vi "PH_Sequencer.PC CheckTOs.vi"(0 "i ref in":refnum<vi>, 5 "error in (no error)":errorcluster) -> (14 "i ref out":refnum<vi>, 19 "error out":errorcluster)   [LabVIEW 2014, in "PH_Sequencer.lvlib"]
doc: "This VI checks whether a timeout occured. It writes this information to own attributes and indicates it on the GUI."
uses:
  PH_Sequencer.lvlib
  PH_Basics/PH_PowerUnit_BaseClass/PH_PowerUnit_BaseClass.SM States.ctl
  PH_Basics/PH_Common/PH_Common.lvlib
  PH_Basics/PH_PowerUnit_BaseClass/PH_PowerUnit_BaseClass.lvlib
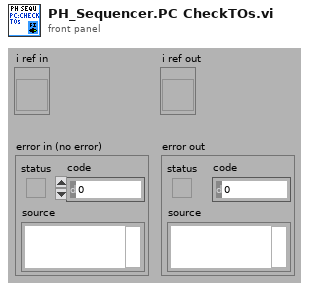
[diagram p1: front panel]
types:
  T1 = typedef "PH_Sequencer.lvlib/PH_Sequencer.i attribute.ctl" = cluster{"GUI Refs":cluster{"Main Off":refnum<vi>, "Fire":refnum<vi>, "Status":refnum<vi>, "Ready":refnum<vi>, "Waiting Time":refnum<vi>, "Timeout":refnum<vi>, "PPMA Ready":refnum<vi>, "Sequencer SM State":refnum<vi>, "PPPA Ready":refnum<vi>, "Calorimeter":refnum<vi>, "Beamline Ready":refnum<vi>, "Clear Beamline":refnum<vi>, "Linkage PPMA Rods":refnum<vi>, "Linkage Current PA":refnum<vi>, "Linkage Current MA":refnum<vi>, "Timing Ready":refnum<vi>, "State Timing":refnum<vi>, "Force Timing":refnum<vi>, "PSDB Shot Comment":refnum<vi>, "State PA Backreflection":refnum<vi>, "Beamline Z6 Ready":refnum<vi>, "Clear Z6 Beamline":refnum<vi>, "Sequence length":refnum<vi>, "Timing Mode":refnum<vi>, "Slow Trigger Settings":refnum<vi>, "Experiment Description":refnum<vi>, "State PSDB":refnum<vi>, "PSDB Ready":refnum<vi>, "Set PSDB Settings":refnum<vi>, "Get PSDB Info":refnum<vi>, "Take Snapshot":refnum<vi>, "Shottype":refnum<vi>, "Experiment":refnum<vi>, "Phase Frontends":refnum<vi>, "PP 45mm PILC in use":refnum<vi>}, "Status Info":cluster{"Machine Status":T2, "WaitingTime":i32, "Timeout":bool}, "Readyness":cluster{"Ready to shot":bool, "PPMA Ready":bool, "PPPA Ready":bool, "BL Ready":bool, "Timing Ready":bool, "BL Z6 Ready":bool, "PSDBReady":bool}, "Instancenames":cluster{"PPMA Rods":string, "PP Current Meas":string, "PH Beamline Chief":string, "PA Backrefl Meas":string, "Z6 Beamline Chief":string}, "Data to read":bool, "Calorimeter":cluster{"Instancename":string, "On":bool, "linked":bool}, "Linkage":cluster{"PPMA Rods":bool, "PP Current Meas":bool, "PHELIX Beamline Chief":bool, "PA Backrefl Meas":bool, "Z6 Beamline Chief":bool}, "Timing":cluster{"Instance":string, "linked":bool, "Status":T2, "Timing Mode":T3, "Slow Trigger Settings":T4, "Info available":cluster{"ext SlowTrigger":bool, "T2":bool, "Mode":bool, "Delay Slow Trigger":bool, "Phase FEs":bool}, "FE Phase":T5}, "Service ID R2S":i32, "PSDB":cluster{"Controller Instance":string, "Controller Status":T2, "Controller linked":bool, "Settings acknowledged":bool, "Current Experiment ID":i16, "Current Shot Type":i16, "Current Comment":string, "Remember Settings":bool, "Write 2 early":bool}, "PSDB Data":cluster{"Main Off?":bool, "Sequence Length":dbl, "Sequence startet":timestamp}, "6P 4Q Positions":cluster{"Instancename":string, "linked":bool, "Position":T6}[], "PUs":T7[]}
  T2 = typedef "PH_StatusHandler.lvlib/PH_StatusHandler.Status.ctl" = i16
  T3 = typedef "PH_Timing.lvlib/PH_Timing.Timing Mode.ctl" = cluster{"T2":i16, "Modeselector":enum32{"10 Hz", "0.5 Hz", "Shot"}}
  T4 = typedef "PH_Timing.lvlib/PH_Timing.Slow Trigger Settings.ctl" = cluster{"Delay":dbl, "externally triggered?":bool}
  T5 = typedef "PH_Timing.lvlib/PH_Timing.Phase FEs.ctl" = cluster{"Phase":dbl}
  T6 = typedef "PH_4_Pos_Selector.lvlib/PH_4_Pos_Selector.Position Selector.ctl" = u16
  T7 = typedef "PH_Sequencer.lvlib/PH_Sequencer.Head.ctl" = cluster{"PowerUnit":T8, "GUI Ref":refnum<vi>, "Information":T9, "linked?":bool, "GUI Ref Current Voltage":refnum<vi>}
  T8 = typedef "PH_PP_Common.lvlib/PH_PP_Common.PUs.ctl" = enum16{"no Info", "PA-19mm-1", "PA-19mm-2", "PA-45mm-PILC", "PA-45mm-MAIN", "MA-PU-1", "MA-PU-2", "MA-PU-3", "MA-PU-4", "MA-PU-5", "MA-PU-6", "MA-FR", "MA-PILC", "PA-45mm-DP"}
  T9 = typedef "PH_Sequencer.lvlib/PH_Sequencer.PU Information.ctl" = cluster{"State":T2, "Waiting Time [s]":dbl, "PU State SM":T10, "PU Timeout SM":T10}
  T10 = typedef "PH_PowerUnit_BaseClass.lvlib/PH_PowerUnit_BaseClass.SM States.ctl" = enum16{".", "Stand by", "Switch PU on", "Configure", "Set Default Voltage", "Set STANDBY", "Set READY", "Wait for Shot Cmd", "Open Dump Rods", "Open Ross Relais", "Close Ross Relais", "Switch PSU on", "Switch PSU off", "Charge", "Switch GD Channel on", "Close Dump Rods", "Rods-TO", "RR-TO", "PSU-TO", "Trigger-TO"}
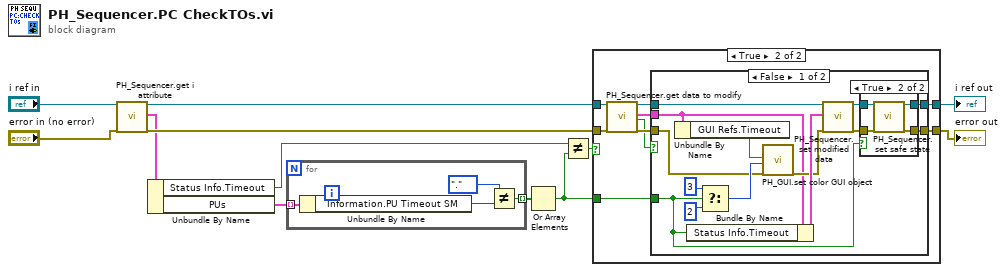
[diagram p0: block diagram]
diagram:
  n1 = call "PH_Sequencer.get i attribute.vi"("i ref in"="i ref in", "error in (no error)"="error in (no error)") -> ("i ref out"=w11:refnum<vi>, "i attribute"=w8:T1, "error out"=w9:errorcluster)  [unwired: 15 in]
  n2 = Unbundle By Name(w8) -> ("Status Info.Timeout"=w4:bool, "PUs"=w2:T7[])
  n3 = for {
    tunnel: w2 -> [w15] mode=indexing
    tunnel: [w16] -> w1 mode=indexing
    n4 = Unbundle By Name(w15) -> ("Information.PU Timeout SM"=w14:T10)
    n5 = Not Equal?(x=PH_PowerUnit_BaseClass.SM_States.".", y=w14) -> (x != y?=w16:bool)
  }
  n6 = Or Array Elements(Boolean array=w1) -> (logical OR=w3:bool)
  n7 = Not Equal?(x=w4, y=w3) -> (x != y?=w5:bool)
  n8 = case shown="True" w5 {
    tunnel: [w18 w27] -> w12
    tunnel: w11 -> [w18 w26]
    tunnel: [w17 w25] -> w10
    tunnel: w9 -> [w17 w24]
    tunnel: w3 -> [_ w23]
    frame False {
    }
    frame True {
      n9 = call "PH_Sequencer.get data to modify.vi"("i ref in"=w26, "error in (no error)"=w24) -> ("i ref out"=w21:refnum<vi>, "i attribute"=w20:T1, "timed out"=w19:bool, "error out"=w22:errorcluster)  [unwired: 14 in]
      n10 = case shown="False" w19 {
        tunnel: [w41 w49] -> w27
        tunnel: [w40 w48] -> w25
        tunnel: w23 -> [w35 _]
        tunnel: w22 -> [w31 w48]
        tunnel: w21 -> [w30 w49]
        tunnel: w20 -> [w29 _]
        frame False {
          n11 = Unbundle By Name(w29) -> ("GUI Refs.Timeout"=w28:refnum<vi>)
          n12 = Bundle By Name(cluster=w29, "Status Info.Timeout"=w35) -> (w39:T1)
          n13 = Select(t=3, s=w35, f=2) -> (s? t:f=w34:i32)
          n14 = call "PH_GUI.set color GUI object.vi"("GUI object Ref"=w28, "State"=w34, "error in (no error)"=w31) -> ("error out"=w33:errorcluster)  [unwired: 16 in]
          n15 = call "PH_Sequencer.set modified data.vi"("i ref in"=w30, "i attribute"=w39, "error in (no error)"=w33) -> ("i ref out"=w38:refnum<vi>, "error out"=w37:errorcluster)  [unwired: 15 in]
          n16 = case shown="True" w35 {
            tunnel: w38 -> [w43 w44]
            tunnel: [w43 w47] -> w41
            tunnel: w37 -> [w42 w46]
            tunnel: [w42 w45] -> w40
            frame False {
            }
            frame True {
              n17 = call "PH_Sequencer.set safe state.vi"("i ref in"=w44, "error in (no error)"=w46) -> ("i ref out"=w47:refnum<vi>, "error out"=w45:errorcluster)  [unwired: 16 in]
            }
          }
        }
        frame True {
        }
      }
    }
  }
  "i ref out" <- w12
  "error out" <- w10
